vi "ini_cluster_read.vi"(8 "error in (no error)":errorcluster caption="错误输入（无错误）", 10 "INI Fomatted Cluster Type":variant, 11 "configuration file path":path caption="配置文件的路径") -> (0 "error out":errorcluster caption="错误输出", 3 "ini cluster out":variant)   [LabVIEW 2011]
uses:
  <vilib>/Utility/config.llb/NI_LVConfig.lvlib
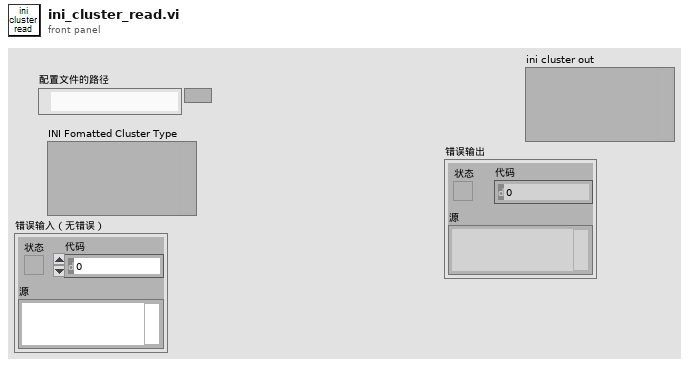
[diagram p1: front panel]
types:
  T1 = typedef "NI_LVConfig.lvlib/Config Data RefNum.ctl" = refnum<k1>
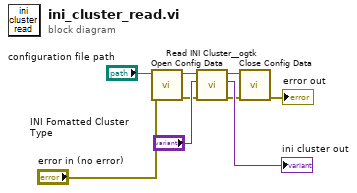
[diagram p0: block diagram]
diagram:
  n1 = call <vilib>:"Open Config Data.vi"("error in (no error)"="error in (no error)", "configuration file path"="configuration file path") -> ("error out"=w4:errorcluster, "refnum"=w9:T1)  [unwired: 7 in, 1 out]
  n2 = call <userlib>:"Read INI Cluster__ogtk.vi"("error in (no error)"=w4, "INI Fomatted Cluster Type"="INI Fomatted Cluster Type", "refnum"=w9) -> ("error out"=w3:errorcluster, "INI Fomatted Cluster"=→"ini cluster out":variant, "dup refnum"=w7:T1)  [unwired: 4 in, 2 out]
  n3 = call <vilib>:"Close Config Data.vi"("error in (no error)"=w3, "refnum"=w7) -> ("error out"=→"error out":errorcluster)  [unwired: 8 in, 1 out]
